vi "Call_C.vi"(8 "Error in (no error)":errorcluster, 9 "Parameters":T2={"RedBall"={"Rmin"=160.0, "Rmax"=255.0, "Gmin"=0.0, "Gmax"=160.0, "Bmin"=0.0, "Bmax"=160.0}, "YellowBall"={"Rmin"=140.0, "Rmax"=255.0, "Gmin"=140.0, "Gmax"=255.0, "Bmin"=0.0, "Bmax"=175.0}, "WhiteBall"={"Rmin"=100.0, "Rmax"=255.0, "Gmin"=100.0, "Gmax"=255.0, "Bmin"=100.0, "Bmax"=255.0}, "BlueBG"={"Rmin"=39.0, "Rmax"=62.0, "Gmin"=91.0, "Gmax"=116.0, "Bmin"=202.0, "Bmax"=255.0}, "BallDiameter"=11.0}, 10 "BillardBox":T1, 11 "Path to PNG file":path) -> (0 "Error out":errorcluster, 1 "Balls coordinates":T4, 3 "Image data":T3)   [LabVIEW 2019]
doc: "Call_C.vi\nCreate Pixmap.bin from PNG file, call Pix2Pos.exe and return coordinates of balls written in Pos.txt in a cluster. \nInput : -Path to PNG file\n -BillardBox containing the coordinates of the billard box\n -Parameters containing all 29 parameters\n -Error in\nOutput : -Balls coordinates containing coordinates and score of each balls\n -Image data containing information of PNG file to print the image in Billard2020\n -Error out"
uses:
  <vilib>/picture/picture.llb/imagedata.ctl
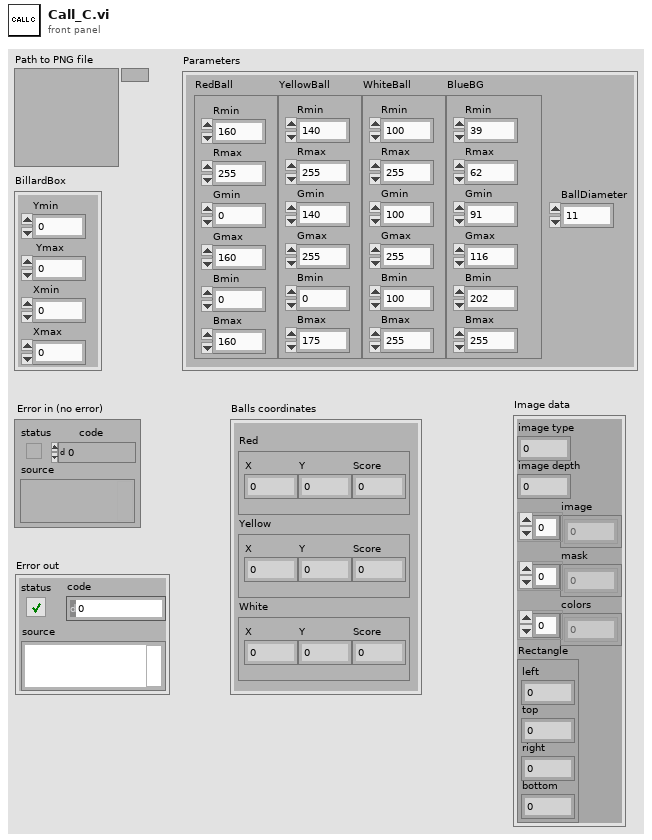
[diagram p1: front panel]
types:
  T1 = cluster{"Ymin":dbl, " Ymax":dbl, "Xmin":dbl, "Xmax":dbl}
  T2 = cluster{"RedBall":cluster{"Rmin":dbl, "Rmax":dbl, "Gmin":dbl, "Gmax":dbl, "Bmin":dbl, "Bmax":dbl}, "YellowBall":cluster{"Rmin":dbl, "Rmax":dbl, "Gmin":dbl, "Gmax":dbl, "Bmin":dbl, "Bmax":dbl}, "WhiteBall":cluster{"Rmin":dbl, "Rmax":dbl, "Gmin":dbl, "Gmax":dbl, "Bmin":dbl, "Bmax":dbl}, "BlueBG":cluster{"Rmin":dbl, "Rmax":dbl, "Gmin":dbl, "Gmax":dbl, "Bmin":dbl, "Bmax":dbl}, "BallDiameter":dbl}
  T3 = typedef "imagedata.ctl" = cluster{"image type":i32, "image depth":i32, "image":u8[], "mask":u8[], "colors":u32[], "Rectangle":cluster{"left":i16, "top":i16, "right":i16, "bottom":i16}}
  T4 = cluster{"Red":cluster{"X":dbl, "Y":dbl, "Score":dbl}, "Yellow":cluster{"X":dbl, "Y":dbl, "Score":dbl}, "White":cluster{"X":dbl, "Y":dbl, "Score":dbl}}
  T5 = enum16{"big-endian, network order", "native, host order", "little-endian"}
  T6 = cluster{"Rmin":dbl, "Rmax":dbl, "Gmin":dbl, "Gmax":dbl, "Bmin":dbl, "Bmax":dbl}
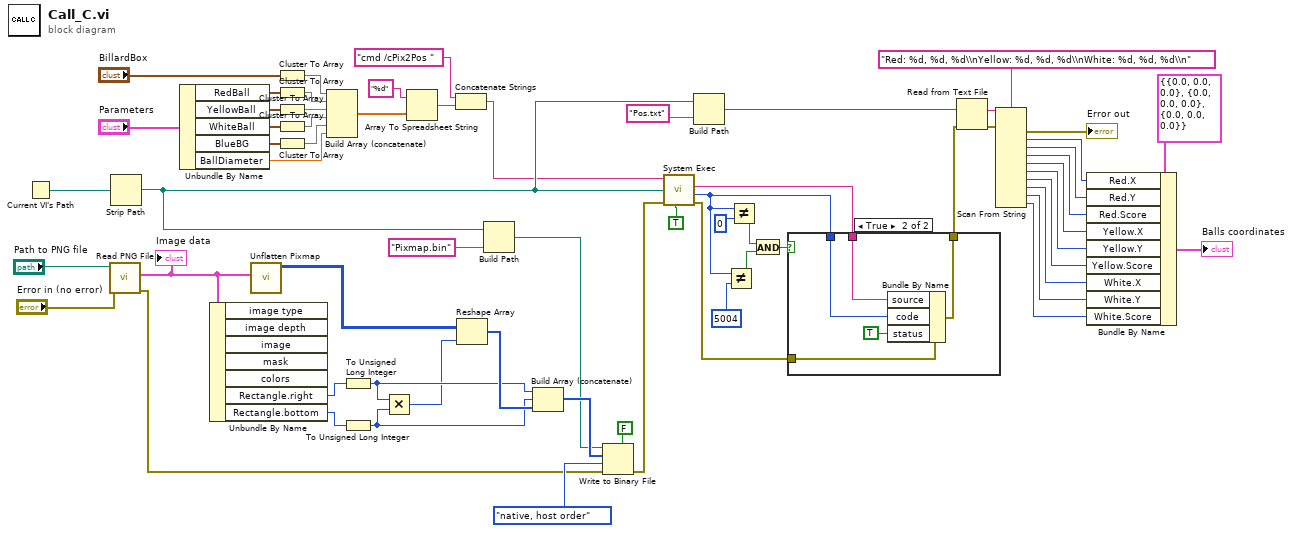
[diagram p0: block diagram]
diagram:
  n1 = Current VI's Path() -> (path=w24:path)
  n2 = call <vilib>:"Read PNG File.vi"("error in (no error)"="Error in (no error)", "path to PNG file"="Path to PNG file") -> ("error out"=w54:errorcluster, "image data"=w26:T3)  [unwired: 7 in, 1 out]
  "Image data" <- w26
  n3 = Strip Path(path=w24) -> (stripped path=w51:path)  [unwired: 1 out]
  n4 = Unbundle By Name("Parameters") -> ("RedBall"=w19:T6, "YellowBall"=w18:T6, "WhiteBall"=w17:T6, "BlueBG"=w16:T6, "BallDiameter"=w15:dbl)
  n5 = Unbundle By Name(w26) -> ("Rectangle.right"=w48:i16, "Rectangle.bottom"=w47:i16)  [unwired: 5 out]
  n6 = call <vilib>:"Unflatten Pixmap.vi"("image data"=w26) -> ("24-bit pixmap"=w63:u32[][])  [unwired: 4 in, 6 out]
  n7 = Cluster To Array(cluster="BillardBox") -> (array=w6:dbl[])
  n8 = Cluster To Array(cluster=w19) -> (array=w10:dbl[])
  n9 = Cluster To Array(cluster=w18) -> (array=w11:dbl[])
  n10 = Cluster To Array(cluster=w17) -> (array=w14:dbl[])
  n11 = Cluster To Array(cluster=w16) -> (array=w13:dbl[])
  n12 = Build Array (concatenate)(w6, w10, w11, w14, w13, w15) -> (w12:dbl[])
  n13 = To Unsigned Long Integer(number=w48) -> (unsigned 32bit integer=w61:u32)
  n14 = To Unsigned Long Integer(number=w47) -> (unsigned 32bit integer=w60:u32)
  n15 = Multiply(x=w61, y=w60) -> (x*y=w59:u32)
  n16 = Array To Spreadsheet String(array=w12, 3:"%d" ("format string")) -> (spreadsheet string=w21:string)  [unwired: 1 in]
  n17 = Concatenate Strings("cmd /cPix2Pos " ("string"), w21) -> (w8:string)
  n18 = Reshape Array(w63, w59) -> (w62:u32[])
  n19 = Build Path(base path=w51, name or relative path="Pixmap.bin") -> (appended path=w53:path)
  n20 = Build Array (concatenate)(w61, w60, w62) -> (w58:u32[])
  n21 = Write to Binary File(file (use dialog)=w53, data=w58, error in=w54, 5:FALSE ("prepend array or string size? (T)"), 9:T5."native, host order" ("byte order (0:big-endian, network order)")) -> (error out=w52:errorcluster)  [unwired: 1 in, 2 out]
  n22 = call <vilib>:"System Exec.vi"("run minimized? (F)"=TRUE, "error in (no error)"=w52, "working directory"=w51, "command line"=w8) -> ("error out"=w30:errorcluster, "return code"=w4:i32, "standard error"=w29:string)  [unwired: 4 in, 1 out]
  n23 = Build Path(base path=w51, name or relative path="Pos.txt") -> (appended path=w27:path)
  n24 = Not Equal?(x=w4, y=5004) -> (x != y?=w1:bool)
  n25 = Not Equal?(x=w4, y=0) -> (x != y?=w2:bool)
  n26 = And(x=w2, y=w1) -> (x .and. y?=w3:bool)
  n27 = case shown="True" w3 {
    tunnel: w29 -> [_ w68]
    tunnel: w30 -> [w64 w69]
    tunnel: w4 -> [_ w67]
    tunnel: [w64 w65] -> w28
    frame False {
    }
    frame True {
      n28 = Bundle By Name(cluster=w69, "source"=w68, "code"=w67, "status"=TRUE) -> (w65:errorcluster)
    }
  }
  n29 = Read from Text File(file (use dialog)=w27, error in=w28) -> (text=w46:string, error out=w31:errorcluster)  [unwired: 2 in, 2 out]
  n30 = Scan From String(format string="Red: %d, %d, %d\\nYellow: %d, %d, %d\\nWhite: %d, %d, %d\\n", input string=w46, error in=w31) -> (error out=→"Error out":errorcluster, output 1=w43:i32, output 2=w42:i32, output 3=w41:i32, output 4=w40:i32, output 5=w39:i32, output 6=w38:i32, output 7=w37:i32, output 8=w36:i32, output 9=w35:i32)  [unwired: 10 in, 2 out]
  n31 = Bundle By Name(cluster=T4 {"Red"={"X"=0.0, "Y"=0.0, "Score"=0.0}, "Yellow"={"X"=0.0, "Y"=0.0, "Score"=0.0}, "White"={"X"=0.0, "Y"=0.0, "Score"=0.0}} ("Balls coordinates 2"), "Red.X"=w43, "Red.Y"=w42, "Red.Score"=w41, "Yellow.X"=w40, "Yellow.Y"=w39, "Yellow.Score"=w38, "White.X"=w37, "White.Y"=w36, "White.Score"=w35) -> (→"Balls coordinates":T4)
